vi "Write to Hardware.vi"(8 "error in":errorcluster, 10 "Values in":dbl[](array[numeric]), 11 "Ballard ARINC-429 Tx Execution Unit in":refnum<class "Ballard ARINC-429 Tx Scheduled Labels Execution Unit.lvclass">) -> (0 "error out":errorcluster, 2 "Values out":dbl[](array[numeric]), 3 "Ballard ARINC-429 Tx Execution Unit out":refnum<class "Ballard ARINC-429 Tx Scheduled Labels Execution Unit.lvclass">)   [LabVIEW 2020, in "Ballard ARINC 429 Engine.lvlib" / "Implementation.lvlib" / "Ballard ARINC-429 Tx Scheduled Labels Execution Unit.lvclass"]
uses:
  Ballard ARINC-429 Tx Scheduled Labels Execution Unit.lvclass
  Ballard ARINC-429 Execution Unit/Ballard ARINC-429 Execution Unit.lvclass
  <instrlib>/BTI429Lib/BTI429LV.lvlib
  C:/Git/niveristand-ballard-arinc429-custom-device/Source/Custom Device Support/Engine/Implementation/Ballard ARINC-429 Execution Unit/Ballard ARINC-429 Execution Unit.lvclass
  C:/Git/niveristand-ballard-arinc429-custom-device/Source/Custom Device Support/Engine/Interfaces/Execution Unit/Execution Unit.lvclass
  C:/Git/niveristand-ballard-arinc429-custom-device/Source/Custom Device Support/Engine/Implementation/Ballard ARINC-429 Tx Execution Unit/Ballard ARINC-429 Tx Scheduled Labels Execution Unit.lvclass
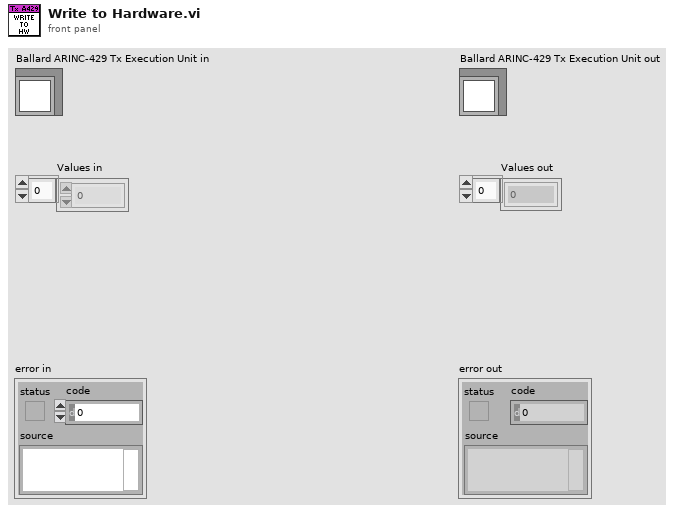
[diagram p1: front panel]
types:
  T1 = typedef "Map of Values Indexes to Channel and Label Indexes.ctl" = map{i32, cluster{"channel index":i32, "label index":i32, "group values start index":i32, "values in group":i32}}
  T2 = typedef "RT Hardware Channel Settings.ctl" = cluster{"channel #":u16, "channel handle":u64, "labels settings for RT":T3[]}
  T3 = typedef "RT Label Settings.ctl" = cluster{"Name":string, "xmlName":string, "label":T4, "transfer period":u32, "SDI_Enabled":bool, "SDI":u8, "parameter driver data":T5, "transfer type":T11, "has timestamp?":bool, "Label Disable/Trigger Channel Reference":T10, "Message Handle":u64, "Initialized?":bool, "Word Initial Raw Value":u32, "Label Timestamp Channel Data Reference":T9, "disabled":bool}
  T4 = typedef "Label.ctl" = u8
  T5 = typedef "RT Parameters.ctl" = cluster{"parameter definitions":T6[], "Rx block data refs":T8[], "Rx values":dbl[], "Tx parameter refs":T10[]}
  T6 = typedef "Parameter Definition.ctl" = cluster{"start index":i32, "size":i32, "encoding":T7, "signed":bool, "scale multiplier":dbl, "scale offset":dbl}
  T7 = typedef "Encoding and Decoding.lvlib/Encoding.ctl" = enum16{"BNR", "BCD", "Discrete"}
  T8 = typedef "Custom Device API.lvlib/Block Data Reference.ctl" = cluster{"Data Reference":T9, "Offset":u64, "Length":u64}
  T9 = typedef "Custom Device API.lvlib/Data Reference.ctl" = i32
  T10 = typedef "Custom Device API.lvlib/Custom Device Item Ref.ctl" = u64
  T11 = typedef "Transfer Type.ctl" = enum16{"Scheduled", "Acyclic", "Block", "Strobe"}
  T12 = typedef "Ballard ARINC 429 Engine.lvlib/Custom Device.lvlib/Hardware Handles.ctl" = cluster{"core handle":u64, "core reader handle":u64, "channel handles":u64[]}
  T13 = cluster{"channel index":i32, "label index":i32, "group values start index":i32, "values in group":i32}
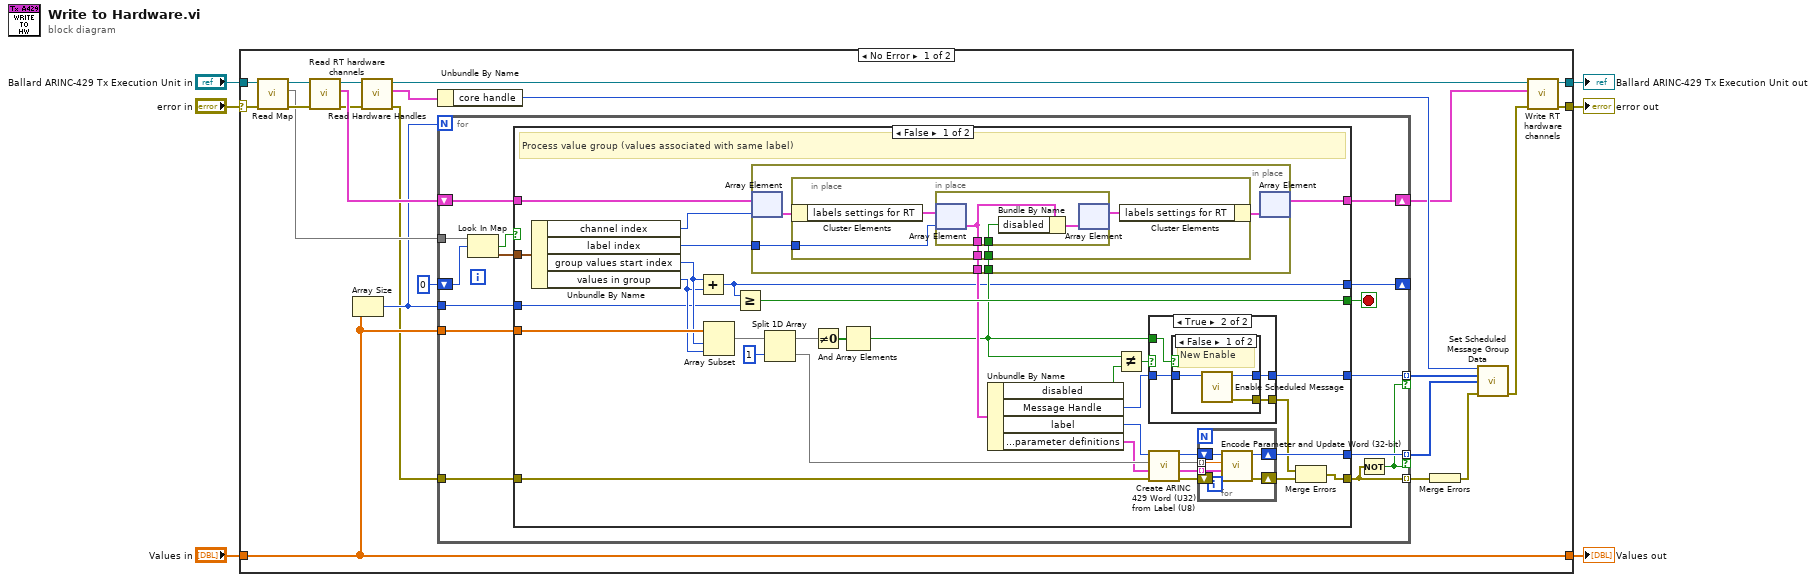
[diagram p0: block diagram]
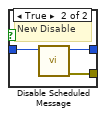
[diagram p3: hidden frame]
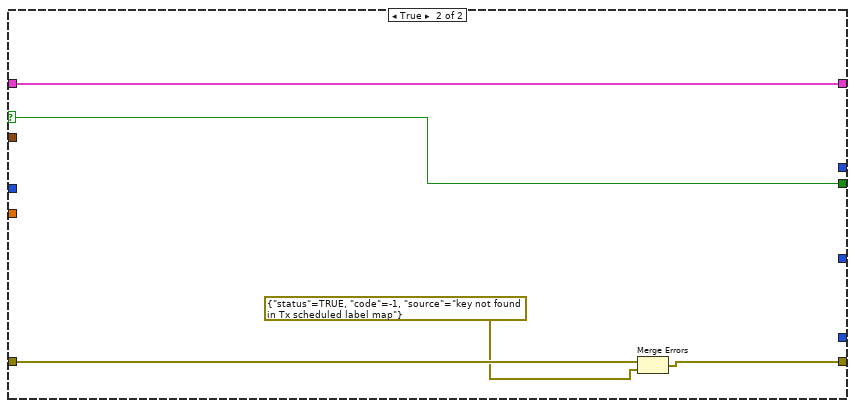
[diagram p4: hidden frame]
diagram:
  n1 = case shown="No Error" "error in" {
    selector: "error in" -> [w21 w110]
    tunnel: [w8 w110] -> w6
    tunnel: [w17 _] -> w4
    tunnel: "Values in" -> [w17 _]
    tunnel: [w9 w111] -> w2
    tunnel: "Ballard ARINC-429 Tx Execution Unit in" -> [w22 w111]
    frame No Error {
      n2 = call "Read Map.vi"("error in"=w21, "Ballard ARINC-429 Tx Execution Unit in"=w22) -> ("error out"=w20:errorcluster, "map from values indexes to RT info indexes"=w19:T1, "Ballard ARINC-429 Tx Execution Unit out"=w23:refnum<class "Ballard ARINC-429 Tx Scheduled Labels Execution Unit.lvclass">)  [unwired: 7 in]
      n3 = call "Read RT hardware channels.vi"("error in"=w20, "Ballard ARINC-429 Tx Execution Unit in"=w23) -> ("error out"=w14:errorcluster, "RT hardware channels"=w25:T2[], "Ballard ARINC-429 Tx Execution Unit out"=w29:refnum<class "Ballard ARINC-429 Tx Scheduled Labels Execution Unit.lvclass">)  [unwired: 7 in]
      n4 = Array Size(array=w17) -> (size(s)=w15:i32)
      n5 = call "Read Hardware Handles.vi"("error in"=w14, "Ballard ARINC-429 Execution Unit in"=w29) -> ("error out"=w13:errorcluster, "hardware handles"=w28:T12, "Ballard ARINC-429 Execution Unit in"=w10:refnum<class "Ballard ARINC-429 Tx Scheduled Labels Execution Unit.lvclass">)  [unwired: 7 in]
      n6 = Unbundle By Name(w28) -> ("core handle"=w27:u64)
      n7 = for {
        N: w15 -> [_]
        tunnel: w17 -> [w37]
        tunnel: [w44] -> w26 mode=indexing if=w31
        tunnel: [w42] -> w24 mode=indexing if=w31
        tunnel: w19 -> [w40]
        shift-right: [w35] -> _
        shift-left: 0 -> [w39]
        tunnel: w15 -> [w36]
        tunnel: w13 -> [w43]
        tunnel: [w32] -> w16 mode=indexing
        shift-right: [w30] -> w11
        shift-left: w25 -> [w41]
        stop <- w33 stop-if-true
        n8 = Look In Map(map=w40, key=w39) -> (key not found?=w34:bool, value=w38:T13)  [unwired: 1 in]
        n9 = case shown="False" w34 {
          selector: w34 -> [_ w106]
          tunnel: [w67 _] -> w44
          tunnel: w43 -> [w74 w109]
          tunnel: [w52 w107] -> w32
          tunnel: [w55 _] -> w42
          tunnel: w41 -> [w47 w105]
          tunnel: w38 -> [w73 _]
          tunnel: w37 -> [w72 _]
          tunnel: w36 -> [w69 _]
          tunnel: [w48 _] -> w35
          tunnel: [w68 w106] -> w33
          tunnel: [w45 w105] -> w30
          frame False {
            # "Process value group (values associated with same label)"
            n10 = Unbundle By Name(w73) -> ("channel index"=w46:i32, "label index"=w49:i32, "group values start index"=w71:i32, "values in group"=w70:i32)
            n11 = Add(x=w71, y=w70) -> (x+y=w48:i32)
            n12 = Array Subset(array=w72, index=w71, length=w70) -> (w65:dbl[])
            n13 = Greater Or Equal?(x=w48, y=w69) -> (x >= y?=w68:bool)
            n14 = Split 1D Array(array=w65, index=1) -> (first subarray=w63:dbl[], second subarray=w64:dbl[])
            n15 = Not Equal To 0?(x=w63) -> (x != 0?=w62:bool[])
            n16 = And Array Elements(Boolean array=w62) -> (logical AND=w50:bool)
            n17 = in-place {
              in-place-border: [w79] -> w51
              in-place-border: w50 -> [w78]
              in-place-border: w49 -> [w77]
              n18 = in-place-array #1(w47, w46) -> (w75:T2)
              n19 = in-place {
                in-place-border: [w84] -> w79
                in-place-border: w78 -> [w83]
                in-place-border: w77 -> [w82]
                n20 = in-place-cluster #2(w75) -> ("labels settings for RT"=w81:T3[])
                n21 = in-place {
                  in-place-border: [w86] -> w84
                  in-place-border: w83 -> [w87]
                  n22 = in-place-array #3(w81, w82) -> (w86:T3)
                  n23 = Bundle By Name(cluster=w86, "disabled"=w87) -> (w85:T3)
                  n24 = in-place-array #3(w85) -> (w80:T3[])  [unwired: 1 out]
                }
                n25 = in-place-cluster #2("labels settings for RT"=w80) -> (w76:T2)
              }
              n26 = in-place-array #1(w76) -> (w45:T2[])  [unwired: 1 out]
            }
            n27 = Unbundle By Name(w51) -> ("disabled"=w57:bool, "Message Handle"=w56:u64, "label"=w60:T4, "parameter driver data.parameter definitions"=w61:T6[])
            n28 = Not Equal?(x=w50, y=w57) -> (x != y?=w58:bool)
            n29 = case shown="True" w58 {
              tunnel: w50 -> [_ w92]
              tunnel: w56 -> [w88 w91]
              tunnel: [w88 w90] -> w55
              tunnel: [_ w89] -> w54
              frame False {
              }
              frame True {
                n30 = case shown="False" w92 {
                  tunnel: w91 -> [w95 w98]
                  tunnel: [w94 w96] -> w89
                  tunnel: [w93 w97] -> w90
                  frame False {
                    # "New Enable"
                    n31 = call <instrlib>:"Enable Scheduled Message.vi"("message handle in"=w95) -> ("error out"=w94:errorcluster, "message handle out"=w93:u64)  [unwired: 9 in]
                  }
                  frame True {
                    # "New Disable"
                    n32 = call <instrlib>:"Disable Scheduled Message.vi"("message handle in"=w98) -> ("error out"=w96:errorcluster, "message handle out"=w97:u64)  [unwired: 9 in]
                  }
                }
              }
            }
            n33 = call "Create ARINC 429 Word (U32) from Label (U8).vi"("label"=w60) -> ("initial word"=w59:u32)  [unwired: 10 in]
            n34 = for {
              tunnel: w64 -> [w104] mode=indexing
              shift-right: [w103] -> w67
              shift-left: w59 -> [w102]
              shift-right: [w100] -> w53
              shift-left: w74 -> [w101]
              tunnel: w61 -> [w99] mode=indexing
              n35 = call "Encode Parameter and Update Word (32-bit).vi"("error in"=w101, "parameter definition"=w99, "parameter value"=w104, "word in"=w102) -> ("error out"=w100:errorcluster, "word out"=w103:u32)  [unwired: 6 in]
            }
            n36 = Merge Errors(w54, w53) -> (w52:errorcluster)
          }
          frame True {
            n37 = Merge Errors(w109, errorcluster {"status"=TRUE, "code"=-1, "source"="key not found in Tx scheduled label map"} ("error in")) -> (w107:errorcluster)
          }
        }
        n38 = Not(x=w32) -> (.not. x?=w31:bool)
      }
      n39 = Merge Errors(w16) -> (w12:errorcluster)
      n40 = call <instrlib>:"Set Scheduled Message Group Data.vi"("core handle in"=w27, "message handles in"=w24, "values"=w26, "error in (no error)"=w12) -> ("error out"=w7:errorcluster)  [unwired: 8 in, 3 out]
      n41 = call "Write RT hardware channels.vi"("error in"=w7, "RT hardware channels"=w11, "Ballard ARINC-429 Tx Execution Unit in"=w10) -> ("error out"=w8:errorcluster, "Ballard ARINC-429 Tx Execution Unit out"=w9:refnum<class "Ballard ARINC-429 Tx Scheduled Labels Execution Unit.lvclass">)  [unwired: 7 in]
    }
    frame Error {
    }
  }
  "error out" <- w6
  "Ballard ARINC-429 Tx Execution Unit out" <- w2
  "Values out" <- w4
